vi "AlliGator Parameter Type to Default Value String.vi"(11 "Parameter Type":string) -> (3 "Default Parameter String":string)   [LabVIEW 2021, in "AlliGator Python Plugins.lvlib"]
doc: "Returns default value of input parameter type."
uses:
  AlliGator Python Plugins.lvlib
panel:
  # "see the AlliGator License on the block diagram (Ctrl+E or Window:Show Block Diagram)"
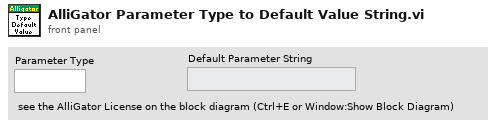
[diagram p1: front panel]
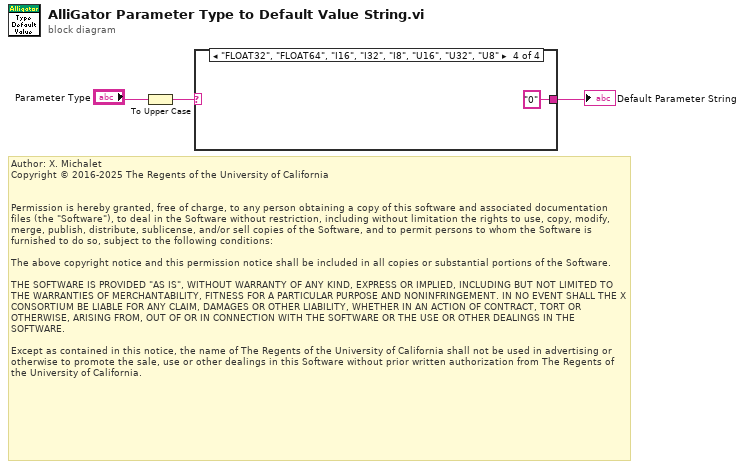
[diagram p0: block diagram]
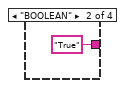
[diagram p3: hidden frame]
diagram:
  # "Author: X. Michalet\nCopyright © 2016-2025 The Regents of the University of California\n \n\nPermission is hereby granted, free of charge, to any person obtaining a copy of this software and associated documentation files (the \"Software\"), to deal in the Software without restriction, including without limitation the rights to use, copy, modify, merge, publish, distribute, sublicense, and/or sell copies of the Software, and to permit persons to whom the Software is furnished to do so, subject to the following conditions:\n\nThe above copyright notice and this permission notice shall be included in all copies or substantial portions of the Software.\n\nTHE SOFTWARE IS PROVIDED \"AS IS\", WITHOUT WARRANTY OF ANY KIND, EXPRESS OR IMPLIED, INCLUDING BUT NOT LIMITED TO THE WARRANTIES OF MERCHANTABILITY, FITNESS FOR A PARTICULAR PURPOSE AND NONINFRINGEMENT. IN NO EVENT SHALL THE X CONSORTIUM BE LIABLE FOR ANY CLAIM, DAMAGES OR OTHER LIABILITY, WHETHER IN AN ACTION OF CONTRACT, TORT OR OTHERWISE, ARISING FROM, OUT OF OR IN CONNECTION WITH THE SOFTWARE OR THE USE OR OTHER DEALINGS IN THE SOFTWARE.\n\nExcept as contained in this notice, the name of The Regents of the University of California shall not be used in advertising or otherwise to promote the sale, use or other dealings in this Software without prior written authorization from The Regents of the University of California."
  n1 = To Upper Case(1:"Parameter Type") -> (0:w1:string)
  n2 = case shown="\"FLOAT32\", \"FLOAT64\", \"I16\", \"I32\", \"I8\", \"U16\", \"U32\", \"U8\"" w1 {
    tunnel: [_ "True" _ "0"] -> w2
    frame "", Default {
    }
    frame "BOOLEAN" {
    }
    frame "PATH", "STRING" {
    }
    frame "FLOAT32", "FLOAT64", "I16", "I32", "I8", "U16", "U32", "U8" {
    }
  }
  "Default Parameter String" <- w2
